vi "core_path_to_lorem_ipsum_database.vi"() -> (0 "path to database":path)   [LabVIEW 2015]
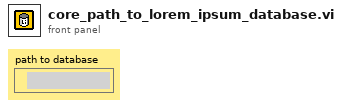
[diagram p1: front panel]
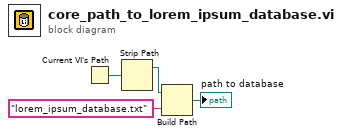
[diagram p0: block diagram]
diagram:
  n1 = Current VI's Path() -> (path=w1:path)
  n2 = Strip Path(path=w1) -> (stripped path=w4:path)  [unwired: 1 out]
  n3 = Build Path(base path=w4, name or relative path="lorem_ipsum_database.txt") -> (appended path=→"path to database":path)
